vi "Simple Controller.vi"() -> ()   [LabVIEW 2011, in "LVH-Leap.lvlib"]
uses:
  vi.lib/LabVIEW Hacker/Leap/LVH-Leap.lvlib
panel:
  out "Leap Connected?":bool
  out "Finger Count per Hand":i32[](array[slide]) scale=0.0..5.0
  in  "stop":bool
  out "Progress of Circle Gestures":dbl[](array[knob]) scale=0.0..10.0
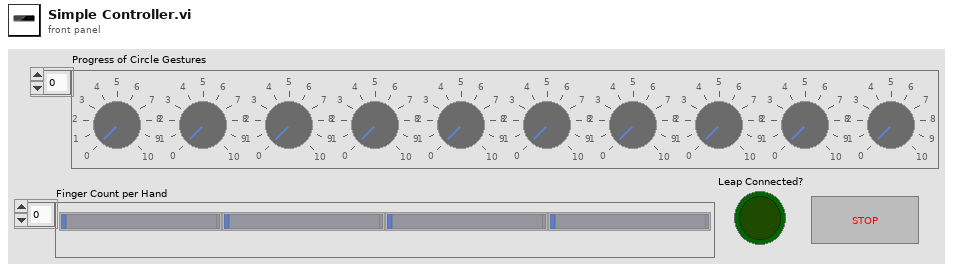
[diagram p1: front panel]
types:
  T1 = typedef "LVH-Leap.lvlib/Leap Handle.ctl" = cluster{"LeapCSharp":refnum<k24>}
  T2 = typedef "LVH-Leap.lvlib/Frame.ctl" = cluster{"ID":i64, "Timestamp":i64, "Hands":T3[], "Key Tap Gestures":T8[], "Screen Tap Gestures":T12[], "Circle Gestures":T13[], "Swipe Gestures":T14[], "Current FPS":dbl}
  T3 = typedef "LVH-Leap.lvlib/Hand.ctl" = cluster{"ID":i32, "Time Visible":sgl, "Direction":T4, "Palm Position":T4, "Palm Position (Stabilized)":T4, "Palm Velocity":T4, "Palm Normal":T4, "Pointables":T5[], "Sphere Radius":sgl, "Sphere Center":T4}
  T4 = typedef "LVH-Leap.lvlib/Vector.ctl" = cluster{"Pitch":sgl, "Yaw":sgl, "Roll":sgl, "Magnitude":sgl, "XYZ":sgl[]}
  T5 = typedef "LVH-Leap.lvlib/Pointable.ctl" = cluster{"ID":i32, "Length":dbl, "Width":dbl, "Time Visible":dbl, "Type":T6, "Direction":T4, "Tip Velocity":T4, "Tip Position":T4, "Tip Position (Stabilized)":T4, "Touch Zone":T7, "Touch Distance":dbl}
  T6 = typedef "LVH-Leap.lvlib/Pointable Type.ctl" = enum16{"Finger", "Tool"}
  T7 = typedef "LVH-Leap.lvlib/Pointable Zone.ctl" = enum16{"None", "Hovering", "Touching"}
  T8 = typedef "LVH-Leap.lvlib/Gesture Key Tap.ctl" = cluster{"Common":T9, "Direction":T4, "Position":T4, "Progress":dbl}
  T9 = typedef "LVH-Leap.lvlib/Gesture Common.ctl" = cluster{"ID":i32, "Duration (s)":dbl, "Gesture Type":T10, "Gesture State":T11}
  T10 = typedef "LVH-Leap.lvlib/Gesture Type.ctl" = enum16{"Invalid", "Swipe", "Circle", "Screen Tap", "Key Tap"}
  T11 = typedef "LVH-Leap.lvlib/Gesture State.ctl" = enum16{"Invalid", "Start", "Update", "Stop"}
  T12 = typedef "LVH-Leap.lvlib/Gesture Screen Tap.ctl" = cluster{"Common":T9, "Direction":T4, "Position":T4, "Progress":dbl}
  T13 = typedef "LVH-Leap.lvlib/Gesture Circle.ctl" = cluster{"Common":T9, "Center":T4, "Normal":T4, "Progress":dbl, "Radius":dbl}
  T14 = typedef "LVH-Leap.lvlib/Gesture Swipe.ctl" = cluster{"Common":T9, "Direction":T4, "Position":T4, "Start Position":T4, "Speed":dbl}
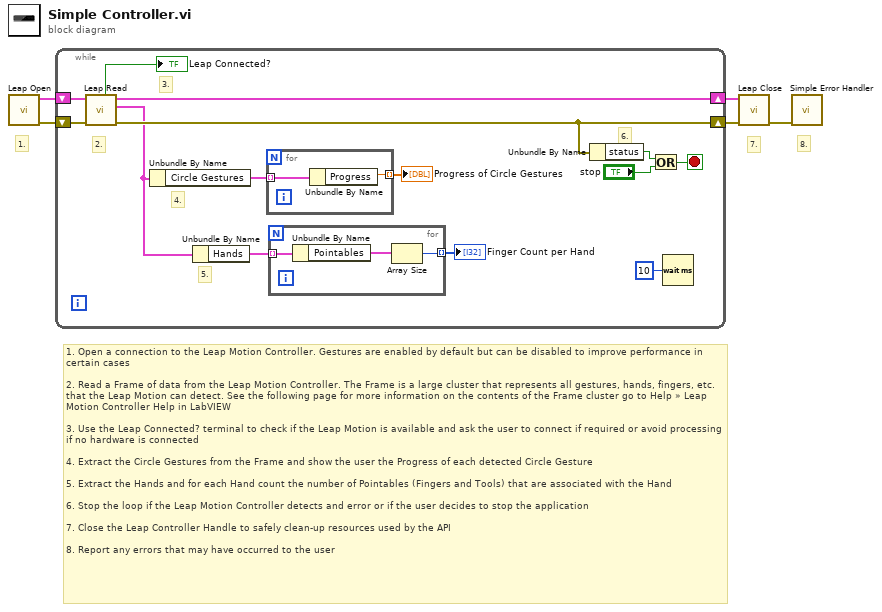
[diagram p0: block diagram]
diagram:
  # "1. Open a connection to the Leap Motion Controller. Gestures are enabled by default but can be disabled to improve performance in certain cases\n\n2. Read a Frame of data from the Leap Motion Controller. The Frame is a large cluster that represents all gestures, hands, fingers, etc. that the Leap Motion can detect. See the following page for more information on the contents of the Frame cluster go to Help » Leap Motion Controller Help in LabVIEW\n\n3. Use the Leap Connected? terminal to check if the Leap Motion is available and ask the user to connect if required or avoid processing if no hardware is connected\n\n4. Extract the Circle Gestures from the Frame and show the user the Progress of each detected Circle Gesture\n\n5. Extract the Hands and for each Hand count the number of Pointables (Fingers and Tools) that are associated with the Hand\n\n6. Stop the loop if the Leap Motion Controller detects and error or if the user decides to stop the application\n\n7. Close the Leap Controller Handle to safely clean-up resources used by the API\n\n8. Report any errors that may have occurred to the user"
  # "8."
  # "7."
  # "1."
  n1 = call "Leap Open.vi"() -> ("error out"=w5:errorcluster, "Leap Handle Out"=w1:T1)  [unwired: 10 in]
  n2 = while {
    shift-right: [w16] -> w3
    shift-left: w5 -> [w18]
    shift-right: [w19] -> w4
    shift-left: w1 -> [w10]
    stop <- w17 stop-if-true
    # "6."
    # "5."
    # "4."
    # "3."
    # "2."
    n3 = call "Leap Read.vi"("error in (no error)"=w18, "Leap Handle In"=w10) -> ("error out"=w16:errorcluster, "Frame"=w15:T2, "Leap Handle Passthrough"=w19:T1, "Leap Connected?"=→"Leap Connected?":bool)  [unwired: 6 in]
    n4 = Unbundle By Name(w15) -> ("Circle Gestures"=w13:T13[])
    n5 = Unbundle By Name(w15) -> ("Hands"=w14:T3[])
    n6 = for {
      tunnel: [w21] -> w11 mode=indexing
      tunnel: w13 -> [w20] mode=indexing
      n7 = Unbundle By Name(w20) -> ("Progress"=w21:dbl)
    }
    "Progress of Circle Gestures" <- w11
    n8 = for {
      tunnel: w14 -> [w24] mode=indexing
      tunnel: [w22] -> w8 mode=indexing
      n9 = Unbundle By Name(w24) -> ("Pointables"=w23:T5[])
      n10 = Array Size(array=w23) -> (size(s)=w22:i32)
    }
    "Finger Count per Hand" <- w8
    n11 = Unbundle By Name(w16) -> ("status"=w6:bool)
    n12 = Or(x=w6, y="stop") -> (x .or. y?=w17:bool)
    n13 = Wait (ms)(milliseconds to wait=u32 10) -> ()  [unwired: 1 out]
  }
  n14 = call "Leap Close.vi"("error in (no error)"=w3, "Leap Handle In"=w4) -> ("error out"=w2:errorcluster)  [unwired: 9 in]
  n15 = call <vilib>:"Simple Error Handler.vi"("error in (no error)"=w2) -> ()  [unwired: 4 in, 5 out]
